vi "User Guided Change Management.vi"() -> ()   [LabVIEW 2025]
panel:
  in  "Add Missing Signals":bool
  in  "Update":bool
  in  "Export Report":bool
  in  "Tree":string(tree)
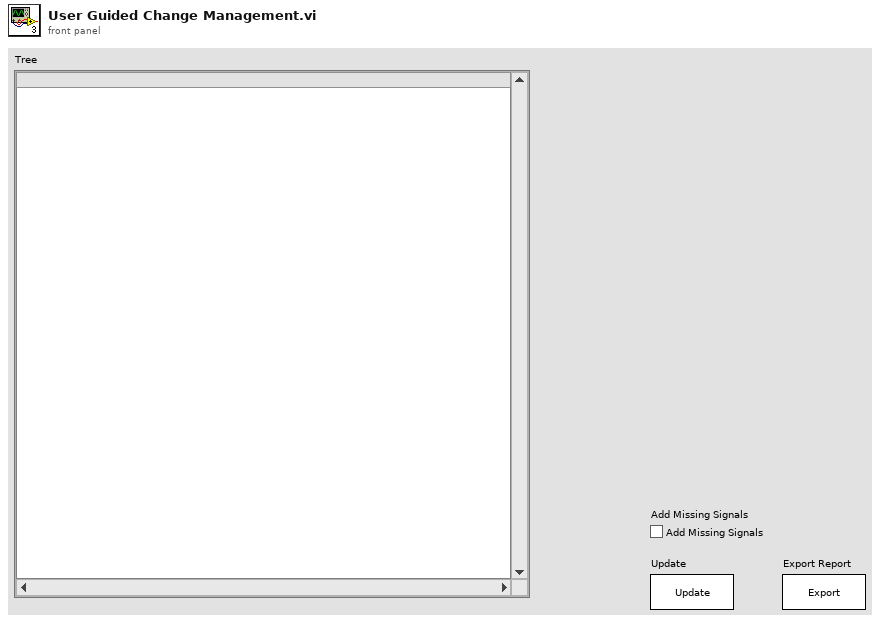
[diagram p1: front panel]
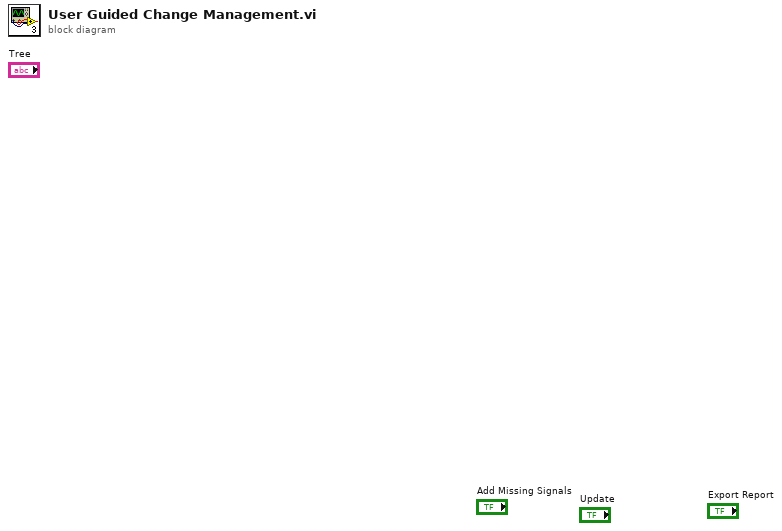
[diagram p0: block diagram]
diagram:
